vi "libssh2_init (Default).vi"(8 "error in (no error)":errorcluster) -> (0 "error out":errorcluster)   [LabVIEW 2013, in "libssh2.lvlib"]
doc: "Initializes libssh2."
uses:
  libssh2.lvlib
  Global Settings.vi
  libssh2.dll
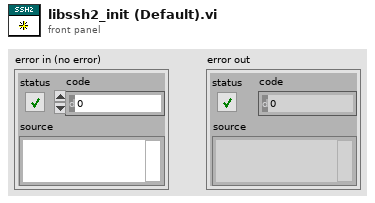
[diagram p1: front panel]
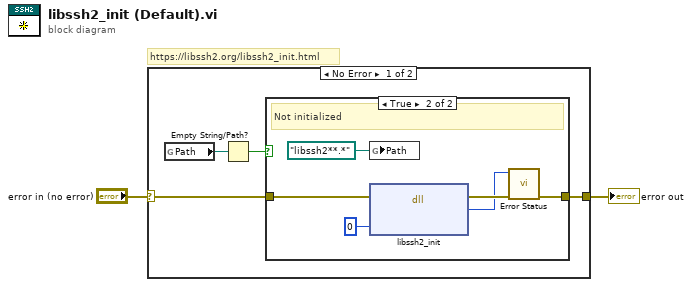
[diagram p0: block diagram]
diagram:
  # "https://libssh2.org/libssh2_init.html"
  n1 = case shown="No Error" "error in (no error)" {
    selector: "error in (no error)" -> [w5 w14]
    tunnel: [w6 w14] -> w2
    frame No Error {
      n2 = global read "Global Settings.vi" "Path"() -> (w3:path)
      n3 = Empty String/Path?(string/path=w3) -> (empty?=w4:bool)
      n4 = case shown="True" w4 {
        tunnel: [w7 w9] -> w6
        tunnel: w5 -> [w7 w11]
        frame False {
          # "Already initialized"
        }
        frame True {
          # "Not initialized"
          n5 = global write "Global Settings.vi" "Path"(path "libssh2**.*") -> ()
          n6 = dll-call lib="C:/Users/pasca/source/repos/libssh2-labview/libssh2/libssh2**.*" fn="libssh2_init"(error in=w11, "flags"=0) -> (error out=w12:errorcluster, "return value"=w8:i32)  [unwired: 3 in, 1 out]
          n7 = call "Error Status.vi"("error in (no error)"=w12, "return value"=w8) -> ("error out"=w9:errorcluster)  [unwired: 9 in]
        }
      }
    }
    frame Error {
    }
  }
  "error out" <- w2
